vi "string2bytearray.vi"(0 "input string":string="1F 0F 50 0A 40 EF 60 3B 01 68 80 01 E8 E6 01 C6 12 0E A6 04 26 07 16 C4 01 77 49 38 01 40 64 18 53 A8 01 00\n1F 0F 50 0A 40 EF 60 3B 01 68 80 01 E8 E6 01 C6 12 0E A6 04 26 07 16 C4 01 77 49 38 01 40 64 18 53 A8 01 00\n1F 0F 50 0A 40 EF 60 3B 01 68 80 01 E8 E6 01 C6 12 0E A6 04 26 07 16 C4 01 77 49 38 01 40 64 18 53 A8 01 00\n1F 0F 50 0A 40 EF 60 3B 01 68 80 01 E8 E6 01 C6 12 0E A6 04 26 07 16 C4 01 77 49 38 01 40 64 18 53 A8 01 00\n") -> (1 "Text Array":string[](array[string]), 2 "Byte array":u16[](array[numeric]) format="%x", 3 "n_bytes":i32)   [LabVIEW 2012]
panel:
  in  "term char":string="00"
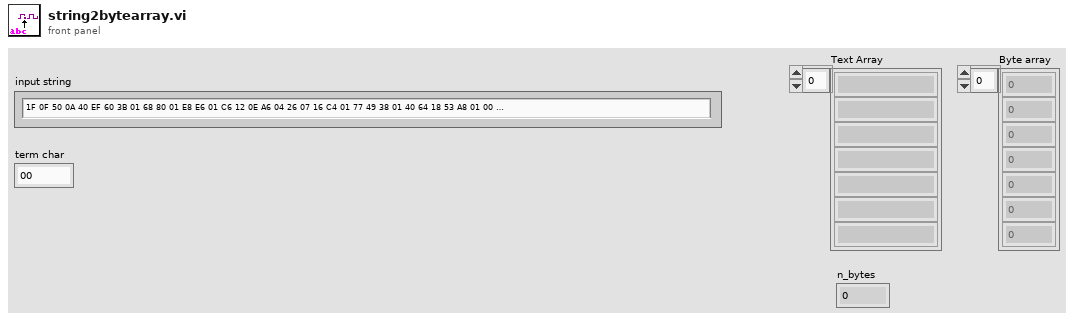
[diagram p1: front panel]
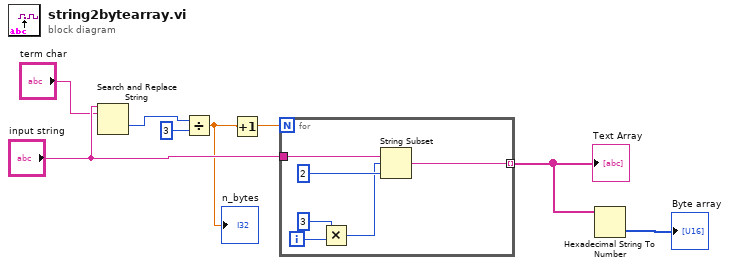
[diagram p0: block diagram]
diagram:
  n1 = Search and Replace String(input string="input string", search string="term char") -> (offset past replacement=w6:i32)  [unwired: 6 in, 3 out]
  n2 = Divide(x=w6, y=3) -> (x/y=w3:dbl)
  "n_bytes" <- w3
  n3 = Increment(x=w3) -> (x+1=w4:dbl)
  n4 = for {
    N: w4 -> [_]
    tunnel: "input string" -> [w14]
    tunnel: [w10] -> w2 mode=indexing
    i -> [w12]
    n5 = Multiply(x=3, y=w12) -> (x*y=w9:i32)
    n6 = String Subset(string=w14, offset (0)=w9, length (rest)=2 ("length (rest)")) -> (substring=w10:string)
  }
  "Text Array" <- w2
  n7 = Hexadecimal String To Number(string=w2) -> (number=→"Byte array":u32[])  [unwired: 2 in, 1 out]
